vi "File_Build Graphic Cluster.vi"(8 "Error":errorcluster, 10 "File Path":path, 11 "Graphic Root Folder":path) -> (0 "Error Out":errorcluster, 3 "Cluster Out":T1)   [LabVIEW 2021]
uses:
  TypeDefs/Cluster_IconFilename.ctl
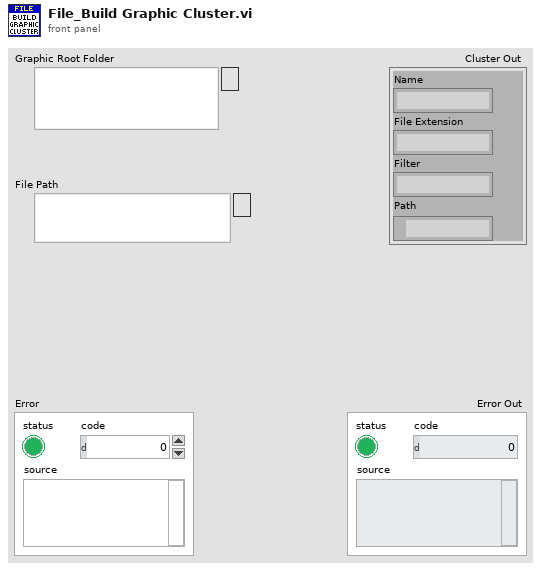
[diagram p1: front panel]
types:
  T1 = typedef "Cluster_IconFilename.ctl" = cluster{"Name":string, "File Extension  ":string, "Filter":string, "Path":path}
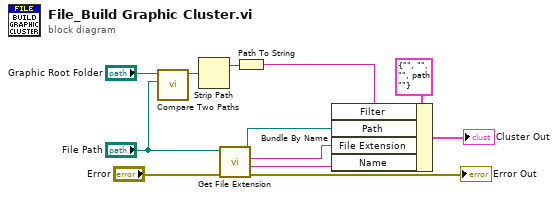
[diagram p0: block diagram]
diagram:
  n1 = call <vilib>:"Compare Two Paths.vi"("Path 2"="File Path", "Path 1"="Graphic Root Folder") -> ("Relative Path from 1 to 2"=w7:path)  [unwired: 1 in, 8 out]
  n2 = Strip Path(path=w7) -> (stripped path=w6:path)  [unwired: 1 out]
  n3 = call <vilib>:"Get File Extension.vi"("error in (no error)"="Error", "file"="File Path") -> ("error out"=→"Error Out":errorcluster, "filename without extension"=w12:string, "lowercase file extension"=w10:string, "dup file"=w2:path)  [unwired: 6 out]
  n4 = Path To String(path=w6) -> (string=w8:string)
  n5 = Bundle By Name(cluster=T1 {"Name"="", "File Extension  "="", "Filter"="", "Path"=path ""}, "Filter"=w8, "Path"=w2, "File Extension"=w10, "Name"=w12) -> (→"Cluster Out":T1)
